vi "Indicator Init.vi"(7 "VolatusAPI":refnum<class "VolatusAPI.lvclass">, 8 "error in (no error)":errorcluster, 10 "JSON":string, 11 "DblNumericStatusIndicator in":refnum<class "DblNumericStatusIndicator.lvclass">) -> (0 "error out":errorcluster, 3 "DblNumericStatusIndicator out":refnum<class "DblNumericStatusIndicator.lvclass">)   [LabVIEW 2020, in "VolatusGUIElements.lvlib" / "DblNumericStatusIndicator.lvclass"]
uses:
  DblNumericStatusIndicator.lvclass
  Volatus/VolatusAPI/VolatusAPI.lvclass
  JSON.ctl
  lv-vecto/Vecto/Group/Group.lvclass
  C:/dev/lv20CE/relink/lv-vecto/Vecto/GroupAbstract/GroupAbstract.lvclass
  DblNumericStatusIndicator.lvclass/DblNumericStatusIndicator.ctl
  c840d708-a4aa-4e42-9474-a77b72826cb9.vi
  <vilib>/JDP Science/JSONtext/JSON text to Variant.vi
  <vilib>/JDP Science/JSONtext/LVClass Serializer/JSONtext LVClass Serializer.lvclass
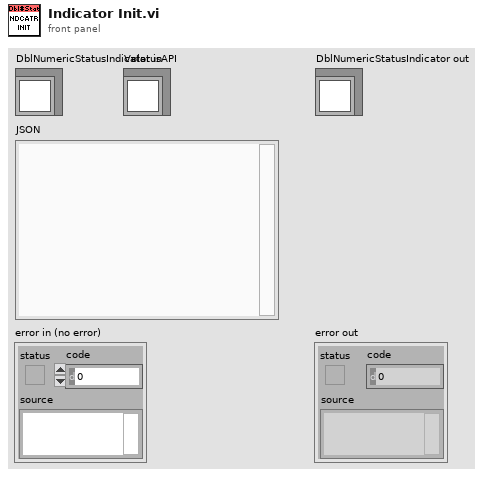
[diagram p1: front panel]
types:
  T1 = typedef "VolatusGUIElements.lvlib/DblNumericStatusIndicator.lvclass/JSON.ctl" = cluster{"Group":string, "Channel":string, "Staleness":dbl}
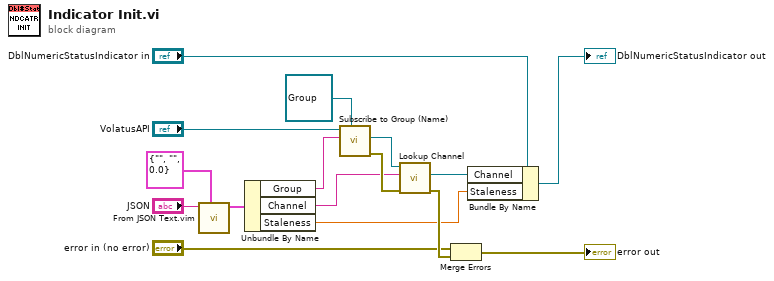
[diagram p0: block diagram]
diagram:
  n1 = call "From JSON Text.vim"("Data Type and Default Value"=T1 {"Group"="", "Channel"="", "Staleness"=0.0} ("JSON"), "JSON"="JSON") -> ("Data out"=w12:T1)  [unwired: 8 in, 1 out]
  n2 = Unbundle By Name(w12) -> ("Group"=w6:string, "Channel"=w5:string, "Staleness"=w4:dbl)
  n3 = call "Subscribe to Group (Name).vi"("Group Type"=refnum<class "Group.lvclass"> refnum ("Group in"), "Group Name"=w6, "VolatusAPI in"="VolatusAPI") -> ("error out"=w11:errorcluster, "Group"=w8:refnum<class "Group.lvclass">)  [unwired: 6 in, 1 out]
  n4 = call "Lookup Channel.vi"("error in (no error)"=w11, "Channel Name"=w5, "Group in"=w8) -> ("error out"=w16:errorcluster, "Channel"=w10:refnum<class "Channel.lvclass">)  [unwired: 6 in, 1 out]
  n5 = Merge Errors("error in (no error)", w16) -> (→"error out":errorcluster)
  n6 = Bundle By Name(cluster="DblNumericStatusIndicator in", "Channel"=w10, "Staleness"=w4) -> (→"DblNumericStatusIndicator out":refnum<class "DblNumericStatusIndicator.lvclass">)
